vi "Info.vi"(8 "error in":errorcluster, 9 "Error to Log":errorcluster, 10 "Message":string, 11 "Logger in":refnum<class "Logger.lvclass">) -> (0 "error out":errorcluster, 3 "Logger out":refnum<class "Logger.lvclass">)   [LabVIEW 2016, in "hse-logger.lvlib" / "Logger.lvclass"]
doc: "Logs an event with level INFO."
uses:
  Logger.lvclass
  LogLevel.ctl
  hse-logger.lvlib
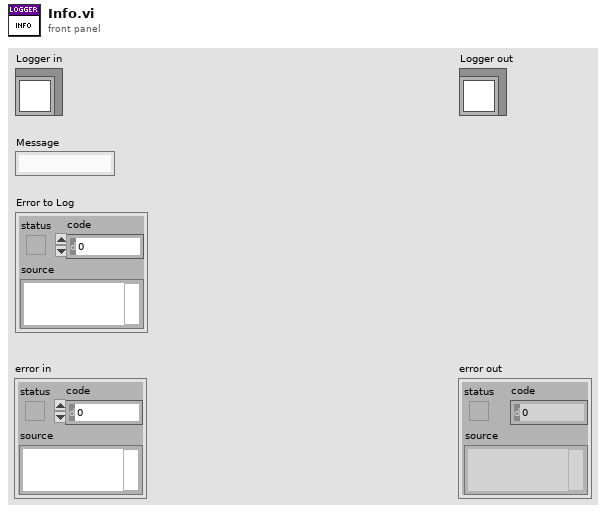
[diagram p1: front panel]
types:
  T1 = typedef "hse-logger.lvlib/LogLevel.ctl" = enum16{"DEBUG", "INFO", "WARNING", "ERROR", "CRITICAL"}
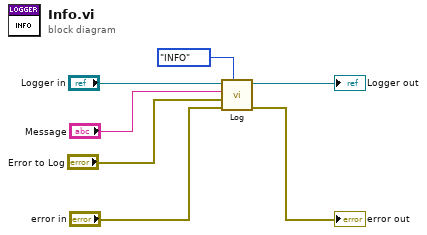
[diagram p0: block diagram]
diagram:
  n1 = call-dynamic "Log.vi"("Level"=LogLevel."INFO", "error in"="error in", "Error to Log"="Error to Log", "Message"="Message", "Logger in"="Logger in") -> ("error out"=→"error out":errorcluster, "Logger out"=→"Logger out":refnum<class "Logger.lvclass">)  [unwired: 5 in]
